vi "salto1.vi"(0 "reference":refnum<vi>) -> ()   [LabVIEW 2015]
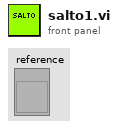
[diagram p1: front panel]
types:
  T1 = enum32{"Bad", "Idle", "Run top level", "Running"}
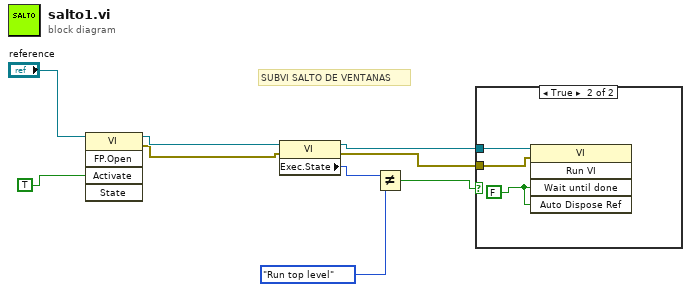
[diagram p0: block diagram]
diagram:
  # "SUBVI SALTO DE VENTANAS"
  n1 = invoke class="VI" method="FP.Open"(reference="reference", "Activate"=TRUE) -> (reference out=w5:refnum<vi>, error out=w4:errorcluster)  [unwired: 3 in, 3 out]
  n2 = property class="VI"(reference=w5, error in=w4) -> (reference out=w7:refnum<vi>, error out=w6:errorcluster, "Exec.State"=w8:T1)
  n3 = Not Equal?(x=w8, y=T1."Run top level") -> (x != y?=w9:bool)
  n4 = case shown="True" w9 {
    tunnel: w7 -> [_ w11]
    tunnel: w6 -> [_ w10]
    frame False {
    }
    frame True {
      w12 = FALSE
      n5 = invoke class="VI" method="Run VI"(reference=w11, error in=w10, "Wait until done"=w12, "Auto Dispose Ref"=w12) -> ()  [unwired: 1 in, 5 out]
    }
  }
